vi "Auto Pickup.vi"() -> (4 "checkpointLiftRaised":bool, 6 "checkpointArmsInPosition":bool, 7 "autoPickupStatus":string, 8 "checkpointPickupArmLocked":bool, 10 "checkpointLiftLowered":bool, 15 "checkpointGrippersClosed":bool)   [LabVIEW 2017]
uses:
  <vilib>/Rock Robotics/WPI/ThirdParty/Phoenix-LabVIEW/Motor Controller/Controls/CTRE_Phoenix_MotorControl_ControlMode.ctl
  <vilib>/Rock Robotics/WPI/Solenoid/WPI_SolenoidValue.ctl
  <vilib>/Rock Robotics/WPI/ThirdParty/Phoenix-LabVIEW/Motor Controller/Get/CTRE_Phoenix_MotorController_GetQuadratureData.vi
  <vilib>/Rock Robotics/WPI/Solenoid/WPI_SolenoidSetEnum.vi
  <vilib>/Rock Robotics/WPI/Solenoid/Deprecated/WPI_SolenoidGetBool.vi
panel:
  out "pickupArmInit":i8
  out "rotateArmInit":i8
  out "pickupArmInPosition":bool
  out "rotateArmInPosition":bool
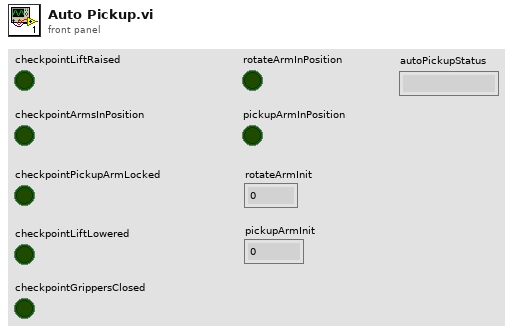
[diagram p1: front panel]
types:
  T1 = typedef "WPI_SolenoidValue.ctl" = enum16{"Off", "On", "Forward", "Reverse"}
  T2 = typedef "WPI_MotorControlDeviceRef.ctl" = cluster{"DeviceStatus":errorcluster, "Type":T3, "PWM":cluster{"PWM Channel":T4, "DeadBand":T5}, "CAN":cluster{"Device Number":u8, "SetOutput VI Ref":variant, "GetOutput VI Ref":variant, "Enable VI Ref":variant, "Disable VI Ref":variant, "Data":variant}, "Invert":bool, "DIO PWM":cluster{"PWM \"Enable\" Channel":T4, "DIOChannel":T6, "PWM Rate":dbl}}
  T3 = typedef "WPI_MotorControlType.ctl" = enum16{"PWM", "CAN", "DIO PWM"}
  T4 = typedef "FPGA_DIOPWMChannel.ctl" = enum8{"PWM 0", "PWM 1", "PWM 2", "PWM 3", "PWM 4", "PWM 5", "PWM 6", "PWM 7", "PWM 8", "PWM 9", "PWM MXP 0", "PWM MXP 1", "PWM MXP 2", "PWM MXP 3", "PWM MXP 4", "PWM MXP 5", "PWM MXP 6", "PWM MXP 7", "PWM MXP 8", "PWM MXP 9", "Invalid"}
  T5 = typedef "WPI_PWMDeadband.ctl" = cluster{"Name":string, "maxPositivePwm":i32, "minPositivePwm":i32, "centerPwm":i32, "maxNegativePwm":i32, "minNegativePwm":i32, "angularRange":u16}
  T6 = typedef "FPGA_DIOChannel.ctl" = enum8{"DIO 0", "DIO 1", "DIO 2", "DIO 3", "DIO 4", "DIO 5", "DIO 6", "DIO 7", "DIO 8", "DIO 9", "DIO MXP 0", "DIO MXP 1", "DIO MXP 2", "DIO MXP 3", "DIO MXP 4", "DIO MXP 5", "DIO MXP 6", "DIO MXP 7", "DIO MXP 8", "DIO MXP 9", "DIO MXP 10", "DIO MXP 11", "DIO MXP 12", "DIO MXP 13", "DIO MXP 14", "DIO MXP 15", "SPI Port CS1", "SPI Port CS2", "SPI Port CS3", "SPI Port MISO", "SPI Port MOSI", "Invalid"}
  T7 = typedef "CTRE_Phoenix_MotorControl_ControlMode.ctl" = u16
  T8 = typedef "WPI_SwitchDevRef.ctl" = cluster{"DevStatus":errorcluster, "DIO Channel":T6, "CntIndex":T9, "Normally Closed":bool}
  T9 = typedef "FPGA_CounterCtrSystemIndex.ctl" = enum8{"Ctr 0", "Ctr 1", "Ctr 2", "Ctr 3", "Ctr 4", "Ctr 5", "Ctr 6", "Ctr 7", "Invalid"}
  T10 = typedef "WPI_EncoderDevRef.ctl" = cluster{"DevStatus":errorcluster, "EncoderIndex":T11, "CounterIndex":T9, "DistancePerCount":dbl, "Decoding Type":T12}
  T11 = typedef "FPGA_EncoderIdx.ctl" = enum8{"Enc 0", "Enc 1", "Enc 2", "Enc 3", "Enc 4", "Enc 5", "Enc 6", "Enc 7", "Invalid"}
  T12 = typedef "WPI_EncoderType.ctl" = enum16{"1x", "2x", "4x"}
  T13 = typedef "WPI_SolenoidDevRef.ctl" = cluster{"DevStatus":errorcluster, "Pneumatics Control Module":u8, "Forward Solenoid Channel":T14, "Reverse Solenoid Channel":T14}
  T14 = typedef "WPI_SolenoidChannel.ctl" = enum8{"Solenoid 0", "Solenoid 1", "Solenoid 2", "Solenoid 3", "Solenoid 4", "Solenoid 5", "Solenoid 6", "Solenoid 7", "Invalid"}
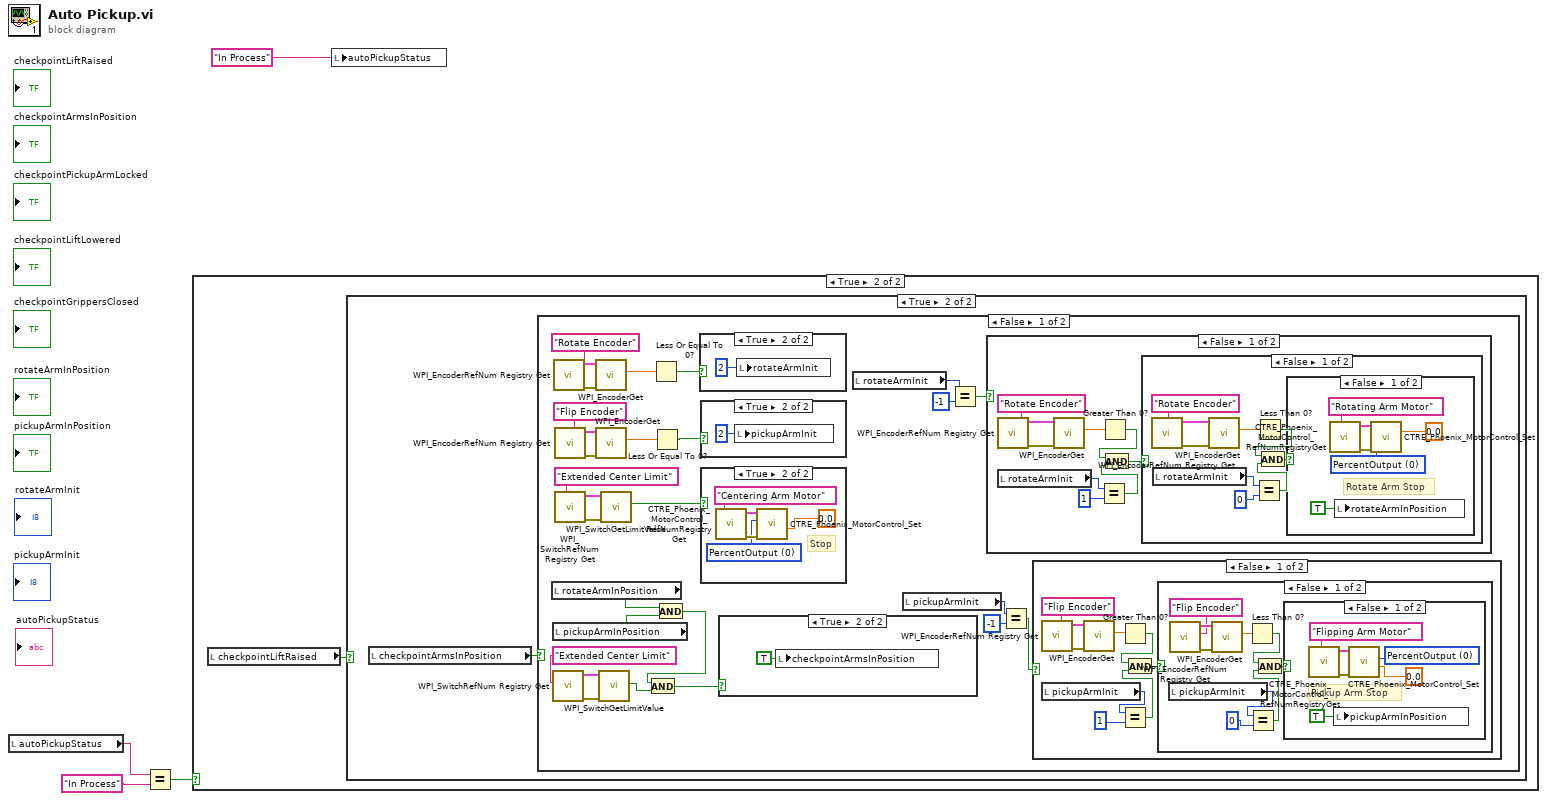
[diagram p0: block diagram]
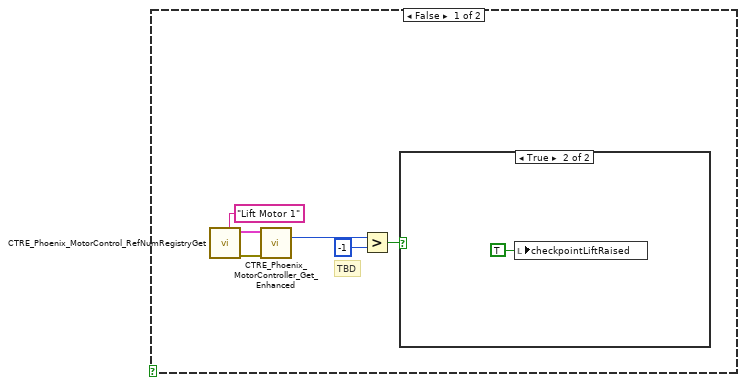
[diagram p3: hidden frame]
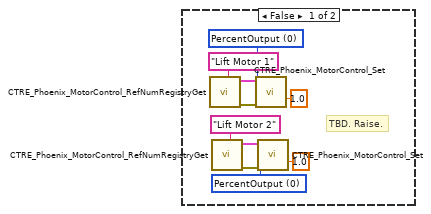
[diagram p4: hidden frame]
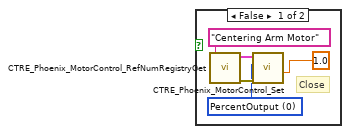
[diagram p6: hidden frame]
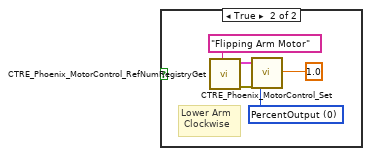
[diagram p7: hidden frame]
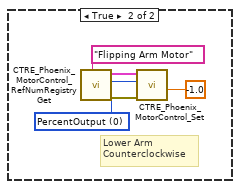
[diagram p8: hidden frame]
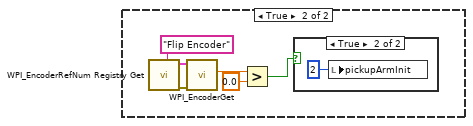
[diagram p9: hidden frame]
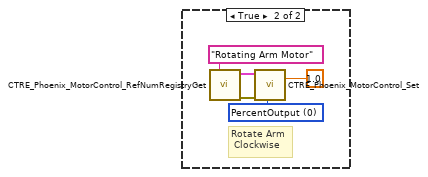
[diagram p11: hidden frame]
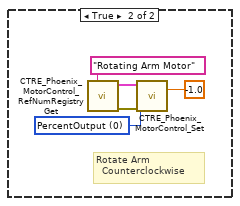
[diagram p12: hidden frame]
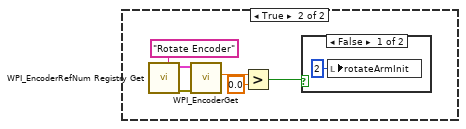
[diagram p13: hidden frame]
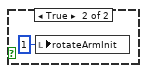
[diagram p14: hidden frame]
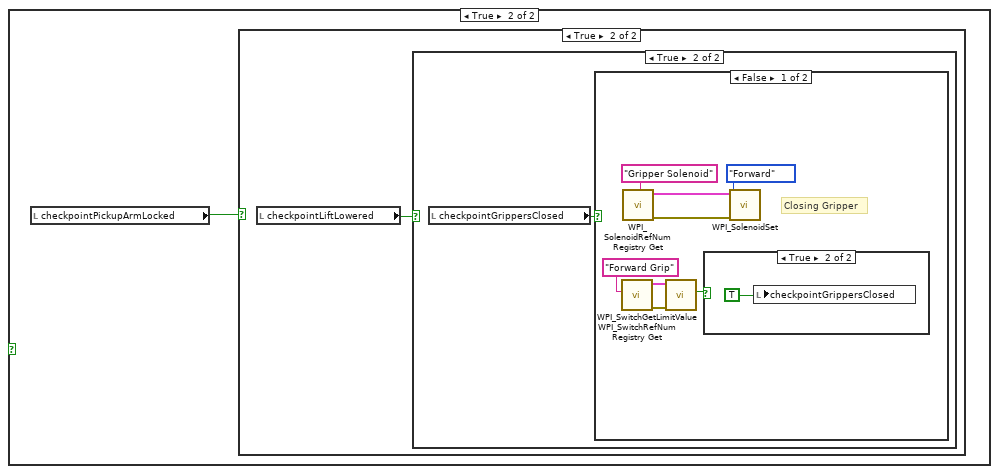
[diagram p17: hidden frame]
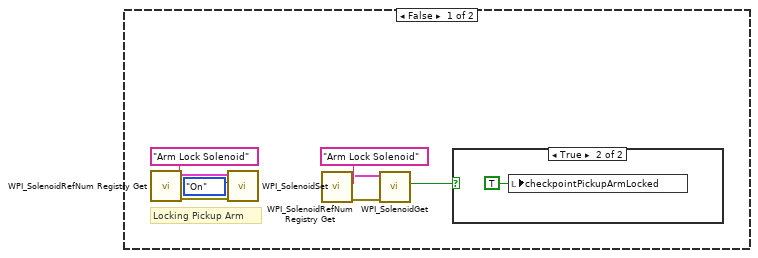
[diagram p18: hidden frame]
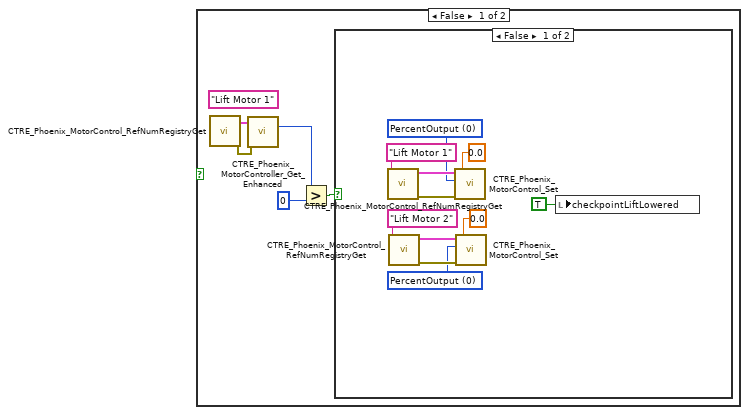
[diagram p20: hidden frame]
diagram:
  n1 = local read "autoPickupStatus"() -> (w2:string)
  n2 = Equal?(x=w2, y="In Process") -> (x = y?=w3:bool)
  n3 = case shown="True" w3 {
    frame False {
    }
    frame True {
      n4 = local read "checkpointLiftRaised"() -> (w5:bool)
      n5 = case shown="True" w5 {
        frame False {
          # "TBD"
          n6 = call <vilib>:"CTRE_Phoenix_MotorControl_RefNumRegistryGet.vi"("refnum name"="Lift Motor 1") -> ("error out"=w10:errorcluster, "PhoenixMotorControlDevRef"=w11:T2)  [unwired: 9 in]
          n7 = call-poly <vilib>:"CTRE_Phoenix_MotorController_Get_Enhanced.vi"("PhoenixMotorControlDevRef"=w11, "error in"=w10) -> ("Quadrature Position"=w8:i32)  [unwired: 10 in, 3 out]
          n8 = Greater?(x=w8, y=-1) -> (0:w6:bool)
          n9 = case shown="True" w6 {
            frame False {
              w12 = T7 0 items=["PercentOutput"=0, "Position"=1, "Velocity"=2, "Current"=3, "Follower"=5, "MotionProfile"=6, "MotionMagic"=7, "MotionMagicArc"=8, "MotionProfileArc"=10, "Disabled"=15] ("Control Mode")
              w13 = T7 0 items=["PercentOutput"=0, "Position"=1, "Velocity"=2, "Current"=3, "Follower"=5, "MotionProfile"=6, "MotionMagic"=7, "MotionMagicArc"=8, "MotionProfileArc"=10, "Disabled"=15] ("Control Mode")
              # "TBD. Raise."
              n10 = call <vilib>:"CTRE_Phoenix_MotorControl_RefNumRegistryGet.vi"("refnum name"="Lift Motor 1") -> ("error out"=w21:errorcluster, "PhoenixMotorControlDevRef"=w20:T2)  [unwired: 9 in]
              n11 = call <vilib>:"CTRE_Phoenix_MotorControl_RefNumRegistryGet.vi"("refnum name"="Lift Motor 2") -> ("error out"=w17:errorcluster, "PhoenixMotorControlDevRef"=w16:T2)  [unwired: 9 in]
              n12 = call <vilib>:"CTRE_Phoenix_MotorControl_Set.vi"("error in (no error)"=w21, "Output"=1.0, "Control Mode"=w13, "PhoenixMotorControlDevRef"=w20) -> ()  [unwired: 6 in, 2 out]
              n13 = call <vilib>:"CTRE_Phoenix_MotorControl_Set.vi"("error in (no error)"=w17, "Output"=1.0, "Control Mode"=w12, "PhoenixMotorControlDevRef"=w16) -> ()  [unwired: 6 in, 2 out]
            }
            frame True {
              n14 = local write "checkpointLiftRaised"(TRUE ("checkpointLiftRaised")) -> ()
            }
          }
        }
        frame True {
          n15 = local read "checkpointArmsInPosition"() -> (w23:bool)
          n16 = case shown="False" w23 {
            frame False {
              n17 = local read "rotateArmInPosition"() -> (w29:bool)
              n18 = local read "pickupArmInPosition"() -> (w28:bool)
              n19 = call <vilib>:"WPI_SwitchRefNum Registry Get.vi"("refnum name"="Extended Center Limit") -> ("error out"=w32:errorcluster, "SwitchDevRef"=w31:T8)  [unwired: 9 in]
              n20 = call <vilib>:"WPI_EncoderRefNum Registry Get.vi"("refnum name"="Rotate Encoder") -> ("error out"=w51:errorcluster, "EncoderDevRef"=w50:T10)  [unwired: 9 in]
              n21 = call <vilib>:"WPI_EncoderRefNum Registry Get.vi"("refnum name"="Flip Encoder") -> ("error out"=w45:errorcluster, "EncoderDevRef"=w44:T10)  [unwired: 9 in]
              n22 = call <vilib>:"WPI_SwitchRefNum Registry Get.vi"("refnum name"="Extended Center Limit") -> ("error out"=w36:errorcluster, "SwitchDevRef"=w35:T8)  [unwired: 9 in]
              n23 = call <vilib>:"WPI_EncoderGet.vi"("error in (no error)"=w51, "EncoderDevRef"=w50) -> ("Distance"=w48:dbl)  [unwired: 4 in, 5 out]
              n24 = call <vilib>:"WPI_EncoderGet.vi"("error in (no error)"=w45, "EncoderDevRef"=w44) -> ("Distance"=w42:dbl)  [unwired: 4 in, 5 out]
              n25 = call <vilib>:"WPI_SwitchGetLimitValue.vi"("error in (no error)"=w32, "SwitchDevRef"=w31) -> ("Switch Pressed"=w30:bool)  [unwired: 7 in, 2 out]
              n26 = call <vilib>:"WPI_SwitchGetLimitValue.vi"("error in (no error)"=w36, "SwitchDevRef"=w35) -> ("Switch Pressed"=w33:bool)  [unwired: 7 in, 2 out]
              n27 = Less Or Equal To 0?(x=w48) -> (x <= 0?=w47:bool)
              n28 = Less Or Equal To 0?(x=w42) -> (x <= 0?=w43:bool)
              n29 = And(x=w29, y=w28) -> (x .and. y?=w27:bool)
              n30 = And(x=w27, y=w30) -> (x .and. y?=w26:bool)
              n31 = case shown="True" w47 {
                frame False {
                }
                frame True {
                  n32 = local write "rotateArmInit"(i8 2 ("rotateArmInit")) -> ()
                }
              }
              n33 = case shown="True" w43 {
                frame False {
                }
                frame True {
                  n34 = local write "pickupArmInit"(i8 2 ("pickupArmInit")) -> ()
                }
              }
              n35 = case shown="True" w33 {
                frame False {
                  w53 = T7 0 items=["PercentOutput"=0, "Position"=1, "Velocity"=2, "Current"=3, "Follower"=5, "MotionProfile"=6, "MotionMagic"=7, "MotionMagicArc"=8, "MotionProfileArc"=10, "Disabled"=15] ("Control Mode")
                  # "Close"
                  n36 = call <vilib>:"CTRE_Phoenix_MotorControl_RefNumRegistryGet.vi"("refnum name"="Centering Arm Motor") -> ("error out"=w56:errorcluster, "PhoenixMotorControlDevRef"=w55:T2)  [unwired: 9 in]
                  n37 = call <vilib>:"CTRE_Phoenix_MotorControl_Set.vi"("error in (no error)"=w56, "Output"=1.0, "Control Mode"=w53, "PhoenixMotorControlDevRef"=w55) -> ()  [unwired: 6 in, 2 out]
                }
                frame True {
                  w58 = T7 0 items=["PercentOutput"=0, "Position"=1, "Velocity"=2, "Current"=3, "Follower"=5, "MotionProfile"=6, "MotionMagic"=7, "MotionMagicArc"=8, "MotionProfileArc"=10, "Disabled"=15] ("Control Mode")
                  # "Stop"
                  n38 = call <vilib>:"CTRE_Phoenix_MotorControl_RefNumRegistryGet.vi"("refnum name"="Centering Arm Motor") -> ("error out"=w61:errorcluster, "PhoenixMotorControlDevRef"=w60:T2)  [unwired: 9 in]
                  n39 = call <vilib>:"CTRE_Phoenix_MotorControl_Set.vi"("error in (no error)"=w61, "Output"=0.0, "Control Mode"=w58, "PhoenixMotorControlDevRef"=w60) -> ()  [unwired: 6 in, 2 out]
                }
              }
              n40 = case shown="True" w26 {
                frame False {
                }
                frame True {
                  n41 = local write "checkpointArmsInPosition"(TRUE ("checkpointArmsInPosition")) -> ()
                }
              }
              n42 = local read "rotateArmInit"() -> (w41:i8)
              n43 = local read "pickupArmInit"() -> (w38:i8)
              n44 = Equal?(x=w41, y=i8 -1) -> (x = y?=w39:bool)
              n45 = case shown="False" w39 {
                frame False {
                  n46 = call <vilib>:"WPI_EncoderRefNum Registry Get.vi"("refnum name"="Rotate Encoder") -> ("error out"=w111:errorcluster, "EncoderDevRef"=w110:T10)  [unwired: 9 in]
                  n47 = local read "rotateArmInit"() -> (w108:i8)
                  n48 = call <vilib>:"WPI_EncoderGet.vi"("error in (no error)"=w111, "EncoderDevRef"=w110) -> ("Distance"=w109:dbl)  [unwired: 4 in, 5 out]
                  n49 = Equal?(x=w108, y=i8 1) -> (x = y?=w105:bool)
                  n50 = Greater Than 0?(x=w109) -> (x > 0?=w106:bool)
                  n51 = And(x=w106, y=w105) -> (x .and. y?=w104:bool)
                  n52 = case shown="False" w104 {
                    frame False {
                      n53 = call <vilib>:"WPI_EncoderRefNum Registry Get.vi"("refnum name"="Rotate Encoder") -> ("error out"=w120:errorcluster, "EncoderDevRef"=w119:T10)  [unwired: 9 in]
                      n54 = local read "rotateArmInit"() -> (w118:i8)
                      n55 = call <vilib>:"WPI_EncoderGet.vi"("error in (no error)"=w120, "EncoderDevRef"=w119) -> ("Distance"=w116:dbl)  [unwired: 4 in, 5 out]
                      n56 = Equal?(x=w118, y=i8 0) -> (x = y?=w115:bool)
                      n57 = Less Than 0?(x=w116) -> (x < 0?=w114:bool)
                      n58 = And(x=w114, y=w115) -> (x .and. y?=w113:bool)
                      n59 = case shown="False" w113 {
                        frame False {
                          w122 = T7 0 items=["PercentOutput"=0, "Position"=1, "Velocity"=2, "Current"=3, "Follower"=5, "MotionProfile"=6, "MotionMagic"=7, "MotionMagicArc"=8, "MotionProfileArc"=10, "Disabled"=15] ("Control Mode")
                          # "Rotate Arm Stop"
                          n60 = call <vilib>:"CTRE_Phoenix_MotorControl_RefNumRegistryGet.vi"("refnum name"="Rotating Arm Motor") -> ("error out"=w125:errorcluster, "PhoenixMotorControlDevRef"=w124:T2)  [unwired: 9 in]
                          n61 = local write "rotateArmInPosition"(TRUE ("rotateArmInPosition")) -> ()
                          n62 = call <vilib>:"CTRE_Phoenix_MotorControl_Set.vi"("error in (no error)"=w125, "Output"=0.0, "Control Mode"=w122, "PhoenixMotorControlDevRef"=w124) -> ()  [unwired: 6 in, 2 out]
                        }
                        frame True {
                          w128 = T7 0 items=["PercentOutput"=0, "Position"=1, "Velocity"=2, "Current"=3, "Follower"=5, "MotionProfile"=6, "MotionMagic"=7, "MotionMagicArc"=8, "MotionProfileArc"=10, "Disabled"=15] ("Control Mode")
                          # "Rotate Arm\n Clockwise"
                          n63 = call <vilib>:"CTRE_Phoenix_MotorControl_RefNumRegistryGet.vi"("refnum name"="Rotating Arm Motor") -> ("error out"=w131:errorcluster, "PhoenixMotorControlDevRef"=w130:T2)  [unwired: 9 in]
                          n64 = call <vilib>:"CTRE_Phoenix_MotorControl_Set.vi"("error in (no error)"=w131, "Output"=1.0, "Control Mode"=w128, "PhoenixMotorControlDevRef"=w130) -> ()  [unwired: 6 in, 2 out]
                        }
                      }
                    }
                    frame True {
                      w133 = T7 0 items=["PercentOutput"=0, "Position"=1, "Velocity"=2, "Current"=3, "Follower"=5, "MotionProfile"=6, "MotionMagic"=7, "MotionMagicArc"=8, "MotionProfileArc"=10, "Disabled"=15] ("Control Mode")
                      # "Rotate Arm\n  Counterclockwise"
                      n65 = call <vilib>:"CTRE_Phoenix_MotorControl_RefNumRegistryGet.vi"("refnum name"="Rotating Arm Motor") -> ("error out"=w136:errorcluster, "PhoenixMotorControlDevRef"=w135:T2)  [unwired: 9 in]
                      n66 = call <vilib>:"CTRE_Phoenix_MotorControl_Set.vi"("error in (no error)"=w136, "Output"=-1.0, "Control Mode"=w133, "PhoenixMotorControlDevRef"=w135) -> ()  [unwired: 6 in, 2 out]
                    }
                  }
                }
                frame True {
                  n67 = call <vilib>:"WPI_EncoderRefNum Registry Get.vi"("refnum name"="Rotate Encoder") -> ("error out"=w142:errorcluster, "EncoderDevRef"=w141:T10)  [unwired: 9 in]
                  n68 = call <vilib>:"WPI_EncoderGet.vi"("error in (no error)"=w142, "EncoderDevRef"=w141) -> ("Distance"=w140:dbl)  [unwired: 4 in, 5 out]
                  n69 = Greater?(x=w140, y=0.0) -> (0:w138:bool)
                  n70 = case shown="False" w138 {
                    frame False {
                      n71 = local write "rotateArmInit"(i8 2 ("rotateArmInit")) -> ()
                    }
                    frame True {
                      n72 = local write "rotateArmInit"(i8 1 ("rotateArmInit")) -> ()
                    }
                  }
                }
              }
              n73 = Equal?(x=w38, y=i8 -1) -> (x = y?=w25:bool)
              n74 = case shown="False" w25 {
                frame False {
                  n75 = call <vilib>:"WPI_EncoderRefNum Registry Get.vi"("refnum name"="Flip Encoder") -> ("error out"=w70:errorcluster, "EncoderDevRef"=w69:T10)  [unwired: 9 in]
                  n76 = local read "pickupArmInit"() -> (w68:i8)
                  n77 = call <vilib>:"WPI_EncoderGet.vi"("error in (no error)"=w70, "EncoderDevRef"=w69) -> ("Distance"=w66:dbl)  [unwired: 4 in, 5 out]
                  n78 = Greater Than 0?(x=w66) -> (x > 0?=w65:bool)
                  n79 = Equal?(x=w68, y=i8 1) -> (x = y?=w64:bool)
                  n80 = And(x=w65, y=w64) -> (x .and. y?=w63:bool)
                  n81 = case shown="False" w63 {
                    frame False {
                      n82 = local read "pickupArmInit"() -> (w77:i8)
                      n83 = call <vilib>:"WPI_EncoderRefNum Registry Get.vi"("refnum name"="Flip Encoder") -> ("error out"=w80:errorcluster, "EncoderDevRef"=w79:T10)  [unwired: 9 in]
                      n84 = call <vilib>:"WPI_EncoderGet.vi"("error in (no error)"=w80, "EncoderDevRef"=w79) -> ("Distance"=w78:dbl)  [unwired: 4 in, 5 out]
                      n85 = Less Than 0?(x=w78) -> (x < 0?=w76:bool)
                      n86 = Equal?(x=w77, y=i8 0) -> (x = y?=w75:bool)
                      n87 = And(x=w76, y=w75) -> (x .and. y?=w74:bool)
                      n88 = case shown="False" w74 {
                        frame False {
                          w81 = T7 0 items=["PercentOutput"=0, "Position"=1, "Velocity"=2, "Current"=3, "Follower"=5, "MotionProfile"=6, "MotionMagic"=7, "MotionMagicArc"=8, "MotionProfileArc"=10, "Disabled"=15] ("Control Mode")
                          # "Pickup Arm Stop"
                          n89 = call <vilib>:"CTRE_Phoenix_MotorControl_RefNumRegistryGet.vi"("refnum name"="Flipping Arm Motor") -> ("error out"=w84:errorcluster, "PhoenixMotorControlDevRef"=w83:T2)  [unwired: 9 in]
                          n90 = local write "pickupArmInPosition"(TRUE ("pickupArmInPosition")) -> ()
                          n91 = call <vilib>:"CTRE_Phoenix_MotorControl_Set.vi"("error in (no error)"=w84, "Output"=0.0, "Control Mode"=w81, "PhoenixMotorControlDevRef"=w83) -> ()  [unwired: 6 in, 2 out]
                        }
                        frame True {
                          w87 = T7 0 items=["PercentOutput"=0, "Position"=1, "Velocity"=2, "Current"=3, "Follower"=5, "MotionProfile"=6, "MotionMagic"=7, "MotionMagicArc"=8, "MotionProfileArc"=10, "Disabled"=15] ("Control Mode")
                          # "Lower Arm\n Clockwise"
                          n92 = call <vilib>:"CTRE_Phoenix_MotorControl_RefNumRegistryGet.vi"("refnum name"="Flipping Arm Motor") -> ("error out"=w90:errorcluster, "PhoenixMotorControlDevRef"=w89:T2)  [unwired: 9 in]
                          n93 = call <vilib>:"CTRE_Phoenix_MotorControl_Set.vi"("error in (no error)"=w90, "Output"=1.0, "Control Mode"=w87, "PhoenixMotorControlDevRef"=w89) -> ()  [unwired: 6 in, 2 out]
                        }
                      }
                    }
                    frame True {
                      w92 = T7 0 items=["PercentOutput"=0, "Position"=1, "Velocity"=2, "Current"=3, "Follower"=5, "MotionProfile"=6, "MotionMagic"=7, "MotionMagicArc"=8, "MotionProfileArc"=10, "Disabled"=15] ("Control Mode")
                      # "Lower Arm\nCounterclockwise"
                      n94 = call <vilib>:"CTRE_Phoenix_MotorControl_RefNumRegistryGet.vi"("refnum name"="Flipping Arm Motor") -> ("error out"=w95:errorcluster, "PhoenixMotorControlDevRef"=w94:T2)  [unwired: 9 in]
                      n95 = call <vilib>:"CTRE_Phoenix_MotorControl_Set.vi"("error in (no error)"=w95, "Output"=-1.0, "Control Mode"=w92, "PhoenixMotorControlDevRef"=w94) -> ()  [unwired: 6 in, 2 out]
                    }
                  }
                }
                frame True {
                  n96 = call <vilib>:"WPI_EncoderRefNum Registry Get.vi"("refnum name"="Flip Encoder") -> ("error out"=w101:errorcluster, "EncoderDevRef"=w100:T10)  [unwired: 9 in]
                  n97 = call <vilib>:"WPI_EncoderGet.vi"("error in (no error)"=w101, "EncoderDevRef"=w100) -> ("Distance"=w99:dbl)  [unwired: 4 in, 5 out]
                  n98 = Greater?(x=w99, y=0.0) -> (0:w97:bool)
                  n99 = case shown="True" w97 {
                    frame False {
                    }
                    frame True {
                      n100 = local write "pickupArmInit"(i8 2 ("pickupArmInit")) -> ()
                    }
                  }
                }
              }
            }
            frame True {
              n101 = local read "checkpointPickupArmLocked"() -> (w148:bool)
              n102 = case shown="True" w148 {
                frame False {
                  # "Locking Pickup Arm"
                  n103 = call <vilib>:"WPI_SolenoidRefNum Registry Get.vi"("refnum name"="Arm Lock Solenoid") -> ("error out"=w155:errorcluster, "SolenoidDevRef"=w154:T13)  [unwired: 9 in]
                  n104 = call-poly <vilib>:"WPI_SolenoidSet.vi"("error in (no error)"=w155, "Value"=WPI_SolenoidValue."On", "SolenoidDevRef"=w154) -> ()  [unwired: 7 in, 2 out]
                  n105 = call <vilib>:"WPI_SolenoidRefNum Registry Get.vi"("refnum name"="Arm Lock Solenoid") -> ("error out"=w151:errorcluster, "SolenoidDevRef"=w150:T13)  [unwired: 9 in]
                  n106 = call-poly <vilib>:"WPI_SolenoidGet.vi"("error in (no error)"=w151, "SolenoidDevRef"=w150) -> ("Value"=w149:bool)  [unwired: 7 in, 2 out]
                  n107 = case shown="True" w149 {
                    frame False {
                    }
                    frame True {
                      n108 = local write "checkpointPickupArmLocked"(TRUE ("checkpointPickupArmLocked")) -> ()
                    }
                  }
                }
                frame True {
                  n109 = local read "checkpointLiftLowered"() -> (w158:bool)
                  n110 = case shown="True" w158 {
                    frame False {
                      (unwired) "Lift Motor 1" ("refnum name")
                      n111 = call <vilib>:"CTRE_Phoenix_MotorControl_RefNumRegistryGet.vi"() -> ("error out"=w161:errorcluster, "PhoenixMotorControlDevRef"=w162:T2)  [unwired: 10 in]
                      n112 = call-poly <vilib>:"CTRE_Phoenix_MotorController_Get_Enhanced.vi"("PhoenixMotorControlDevRef"=w162, "error in"=w161) -> ("Quadrature Position"=w160:i32)  [unwired: 10 in, 3 out]
                      n113 = Greater?(x=w160, y=0) -> (0:w163:bool)
                      n114 = case shown="False" w163 {
                        frame False {
                          w164 = T7 0 items=["PercentOutput"=0, "Position"=1, "Velocity"=2, "Current"=3, "Follower"=5, "MotionProfile"=6, "MotionMagic"=7, "MotionMagicArc"=8, "MotionProfileArc"=10, "Disabled"=15] ("Control Mode")
                          w165 = T7 0 items=["PercentOutput"=0, "Position"=1, "Velocity"=2, "Current"=3, "Follower"=5, "MotionProfile"=6, "MotionMagic"=7, "MotionMagicArc"=8, "MotionProfileArc"=10, "Disabled"=15] ("Control Mode")
                          n115 = call <vilib>:"CTRE_Phoenix_MotorControl_RefNumRegistryGet.vi"("refnum name"="Lift Motor 1") -> ("error out"=w172:errorcluster, "PhoenixMotorControlDevRef"=w171:T2)  [unwired: 9 in]
                          n116 = call <vilib>:"CTRE_Phoenix_MotorControl_RefNumRegistryGet.vi"("refnum name"="Lift Motor 2") -> ("error out"=w168:errorcluster, "PhoenixMotorControlDevRef"=w167:T2)  [unwired: 9 in]
                          n117 = call <vilib>:"CTRE_Phoenix_MotorControl_Set.vi"("error in (no error)"=w172, "Output"=0.0, "Control Mode"=w165, "PhoenixMotorControlDevRef"=w171) -> ()  [unwired: 6 in, 2 out]
                          n118 = call <vilib>:"CTRE_Phoenix_MotorControl_Set.vi"("error in (no error)"=w168, "Output"=0.0, "Control Mode"=w164, "PhoenixMotorControlDevRef"=w167) -> ()  [unwired: 6 in, 2 out]
                          n119 = local write "checkpointLiftLowered"(TRUE ("checkpointLiftLowered")) -> ()
                        }
                        frame True {
                          w175 = T7 0 items=["PercentOutput"=0, "Position"=1, "Velocity"=2, "Current"=3, "Follower"=5, "MotionProfile"=6, "MotionMagic"=7, "MotionMagicArc"=8, "MotionProfileArc"=10, "Disabled"=15] ("Control Mode")
                          w176 = T7 0 items=["PercentOutput"=0, "Position"=1, "Velocity"=2, "Current"=3, "Follower"=5, "MotionProfile"=6, "MotionMagic"=7, "MotionMagicArc"=8, "MotionProfileArc"=10, "Disabled"=15] ("Control Mode")
                          # "Lowering Lift Arm.\nAssuming Negative"
                          n120 = call <vilib>:"CTRE_Phoenix_MotorControl_RefNumRegistryGet.vi"("refnum name"="Lift Motor 1") -> ("error out"=w183:errorcluster, "PhoenixMotorControlDevRef"=w182:T2)  [unwired: 9 in]
                          n121 = call <vilib>:"CTRE_Phoenix_MotorControl_RefNumRegistryGet.vi"("refnum name"="Lift Motor 2") -> ("error out"=w179:errorcluster, "PhoenixMotorControlDevRef"=w178:T2)  [unwired: 9 in]
                          n122 = call <vilib>:"CTRE_Phoenix_MotorControl_Set.vi"("error in (no error)"=w183, "Output"=-1.0, "Control Mode"=w176, "PhoenixMotorControlDevRef"=w182) -> ()  [unwired: 6 in, 2 out]
                          n123 = call <vilib>:"CTRE_Phoenix_MotorControl_Set.vi"("error in (no error)"=w179, "Output"=-1.0, "Control Mode"=w175, "PhoenixMotorControlDevRef"=w178) -> ()  [unwired: 6 in, 2 out]
                        }
                      }
                    }
                    frame True {
                      n124 = local read "checkpointGrippersClosed"() -> (w185:bool)
                      n125 = case shown="False" w185 {
                        frame False {
                          # "Closing Gripper"
                          n126 = call <vilib>:"WPI_SwitchRefNum Registry Get.vi"("refnum name"="Forward Grip") -> ("error out"=w189:errorcluster, "SwitchDevRef"=w188:T8)  [unwired: 9 in]
                          n127 = call <vilib>:"WPI_SolenoidRefNum Registry Get.vi"("refnum name"="Gripper Solenoid") -> ("error out"=w193:errorcluster, "SolenoidDevRef"=w192:T13)  [unwired: 9 in]
                          n128 = call <vilib>:"WPI_SwitchGetLimitValue.vi"("error in (no error)"=w189, "SwitchDevRef"=w188) -> ("Switch Pressed"=w187:bool)  [unwired: 7 in, 2 out]
                          n129 = case shown="True" w187 {
                            frame False {
                            }
                            frame True {
                              n130 = local write "checkpointGrippersClosed"(TRUE ("checkpointGrippersClosed")) -> ()
                            }
                          }
                          n131 = call-poly <vilib>:"WPI_SolenoidSet.vi"("error in (no error)"=w193, "Value"=WPI_SolenoidValue."Forward", "SolenoidDevRef"=w192) -> ()  [unwired: 7 in, 2 out]
                        }
                        frame True {
                          n132 = local write "autoPickupStatus"("Completed" ("autoPickupStatus")) -> ()
                          n133 = local write "pickupArmInPosition"(FALSE ("pickupArmInPosition")) -> ()
                          n134 = local write "rotateArmInPosition"(FALSE ("rotateArmInPosition")) -> ()
                          n135 = local write "checkpointLiftRaised"(FALSE ("checkpointLiftRaised")) -> ()
                          n136 = local write "checkpointArmsInPosition"(FALSE ("checkpointArmsInPosition")) -> ()
                          n137 = local write "checkpointPickupArmLocked"(FALSE ("checkpointPickupArmLocked")) -> ()
                          n138 = local write "checkpointGrippersClosed"(FALSE ("checkpointGrippersClosed")) -> ()
                          n139 = local write "rotateArmInit"(i8 -1 ("rotateArmInit")) -> ()
                          n140 = local write "pickupArmInit"(i8 -1 ("pickupArmInit")) -> ()
                          n141 = local write "checkpointLiftLowered"(FALSE ("checkpointLiftLowered")) -> ()
                        }
                      }
                    }
                  }
                }
              }
            }
          }
        }
      }
    }
  }
  n142 = local write "autoPickupStatus"("In Process" ("autoPickupStatus")) -> ()
